vi "Parse.vi"(8 "error in (no error)":errorcluster, 11 "PathCommands in":refnum<class "PathCommands.lvclass">) -> (0 "error out":errorcluster, 3 "PathCommands out":refnum<class "PathCommands.lvclass">)   [LabVIEW 2019, in "PathCommands.lvclass"]
uses:
  PathCommands.lvclass
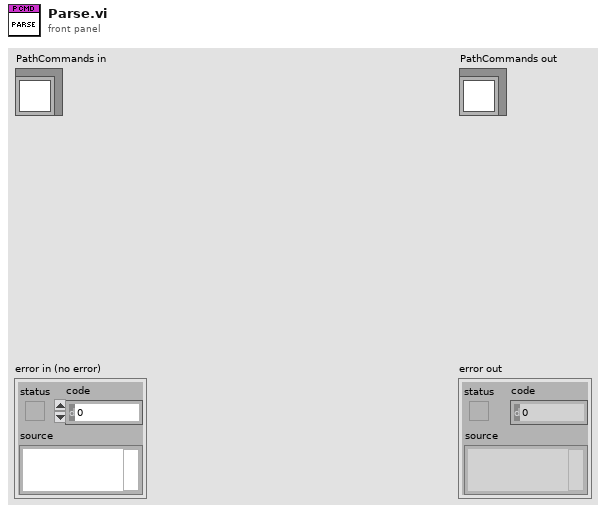
[diagram p1: front panel]
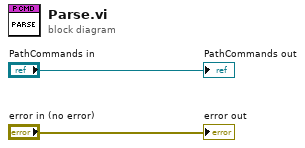
[diagram p0: block diagram]
diagram:
  "error out" <- "error in (no error)"
  "PathCommands out" <- "PathCommands in"
